vi "Instr_SetPrivateData.vi"(8 "error in (no error)":errorcluster, 11 "KE2000 in":refnum<class "KE2000.lvclass">) -> (0 "error out":errorcluster, 3 "KE2000 out":refnum<class "KE2000.lvclass">)   [LabVIEW 2013, in "KE2000.lvclass"]
uses:
  KE2000.lvclass
  InstrumentSetup.vi
  KE2000_CommandsGlobal.vi
  InstrControl.lvclass
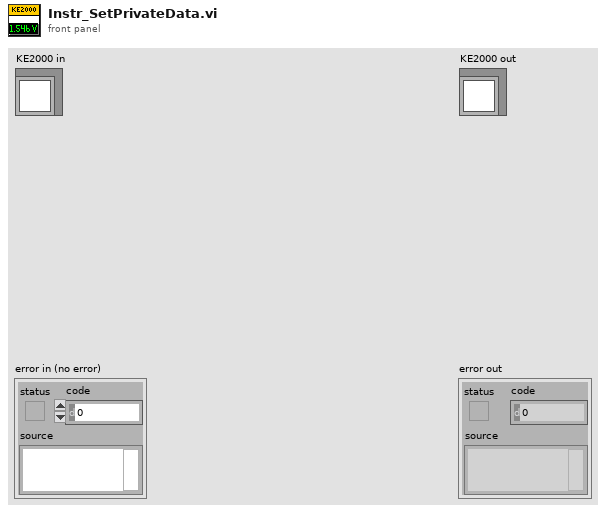
[diagram p1: front panel]
types:
  T1 = cluster{"Range":u16, "Range Value":dbl, "Function":u16, "GPIB Address":string}
  T2 = cluster{"GPIB address":string, "Instrument name":string, "Instrument type":u16, "Command \"Reset\"":string, "Command \"Initialise\"":string, "Command \"Read Data\"":string}
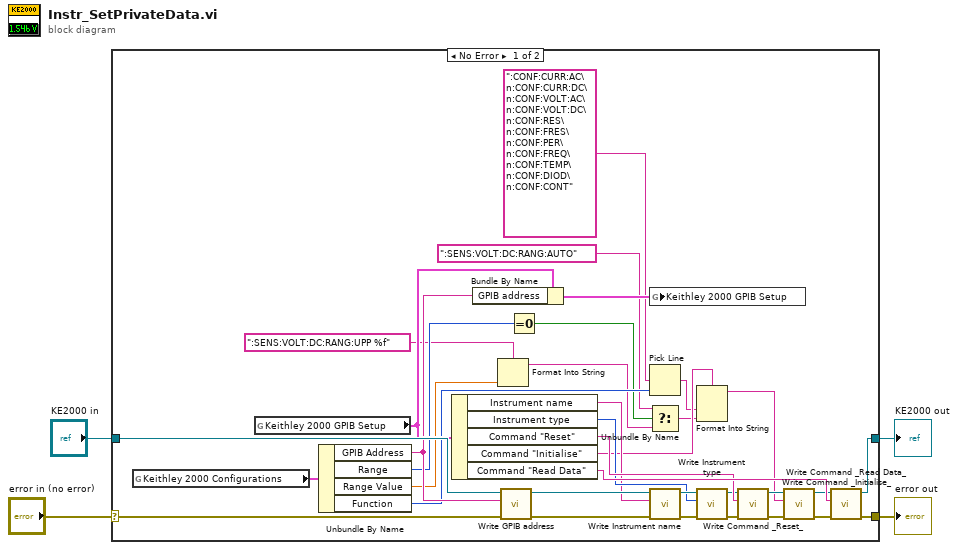
[diagram p0: block diagram]
diagram:
  n1 = case shown="No Error" "error in (no error)" {
    selector: "error in (no error)" -> [w38 w40]
    tunnel: [w24 w40] -> w3
    tunnel: "KE2000 in" -> [w35 w39]
    tunnel: [w21 w39] -> w1
    frame No Error {
      n2 = global read "InstrumentSetup.vi" "Keithley 2000 Configurations"() -> (w33:T1)
      n3 = global read "KE2000_CommandsGlobal.vi" "Keithley 2000 GPIB Setup"() -> (w31:T2)
      n4 = Unbundle By Name(w33) -> ("GPIB Address"=w17:string, "Range"=w11:u16, "Range Value"=w9:dbl, "Function"=w14:u16)
      n5 = Unbundle By Name(w31) -> ("Instrument name"=w18:string, "Instrument type"=w19:u16, "Command \"Reset\""=w29:string, "Command \"Initialise\""=w16:string, "Command \"Read Data\""=w30:string)
      n6 = Bundle By Name(cluster=w31, "GPIB address"=w17) -> (w32:T2)
      n7 = Format Into String(format string=":SENS:VOLT:DC:RANG:UPP %f", w9) -> (resulting string=w8:string)  [unwired: 2 in, 1 out]
      n8 = call-dynamic "Write GPIB address.vi"("error in (no error)"=w38, "GPIB address"=w17, "InstControl in"=w35) -> ("error out"=w37:errorcluster, "InstControl out"=w34:refnum<class "KE2000.lvclass">)  [unwired: 7 in]
      n9 = Equal To 0?(x=w11) -> (x = 0?=w12:bool)
      n10 = global write "KE2000_CommandsGlobal.vi" "Keithley 2000 GPIB Setup"(w32) -> ()
      n11 = Pick Line(multi-line string=":CONF:CURR:AC\n:CONF:CURR:DC\n:CONF:VOLT:AC\n:CONF:VOLT:DC\n:CONF:RES\n:CONF:FRES\n:CONF:PER\n:CONF:FREQ\n:CONF:TEMP\n:CONF:DIOD\n:CONF:CONT", line index=w14) -> (output string=w13:string)  [unwired: 1 in]
      n12 = Select(t=":SENS:VOLT:DC:RANG:AUTO", s=w12, f=w8) -> (s? t:f=w6:string)
      n13 = call-dynamic "Write Instrument name.vi"("error in (no error)"=w37, "Instrument name"=w18, "InstControl in"=w34) -> ("error out"=w36:errorcluster, "InstControl out"=w20:refnum<class "KE2000.lvclass">)  [unwired: 7 in]
      n14 = Format Into String(format string=w16, w13, w6) -> (resulting string=w5:string)  [unwired: 2 in, 1 out]
      n15 = call-dynamic "Write Instrument type.vi"("error in (no error)"=w36, "Instrument type"=w19, "InstControl in"=w20) -> ("error out"=w27:errorcluster, "InstControl out"=w28:refnum<class "KE2000.lvclass">)  [unwired: 7 in]
      n16 = call-dynamic "Write Command _Reset_.vi"("error in (no error)"=w27, "Command \"Reset\""=w29, "MultimeterControl in"=w28) -> ("error out"=w26:errorcluster, "MultimeterControl out"=w23:refnum<class "KE2000.lvclass">)  [unwired: 7 in]
      n17 = call-dynamic "Write Command _Initialise_.vi"("error in (no error)"=w26, "Command \"Initialise\""=w5, "MultimeterControl in"=w23) -> ("error out"=w25:errorcluster, "MultimeterControl out"=w22:refnum<class "KE2000.lvclass">)  [unwired: 7 in]
      n18 = call-dynamic "Write Command _Read Data_.vi"("error in (no error)"=w25, "Command \"Read Data\""=w30, "MultimeterControl in"=w22) -> ("error out"=w24:errorcluster, "MultimeterControl out"=w21:refnum<class "KE2000.lvclass">)  [unwired: 7 in]
    }
    frame Error {
    }
  }
  "error out" <- w3
  "KE2000 out" <- w1
